vi "Get Platform.vi"(11 "Platform":T2) -> (3 "Platform":T1)   [LabVIEW 2011, in "LMH-LINX.lvlib"]
uses:
  LMH-LINX.lvlib
  Type Defs/User Platform.ctl
  Type Defs/Platform.ctl
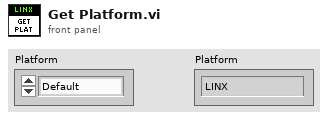
[diagram p1: front panel]
types:
  T1 = typedef "LMH-LINX.lvlib/Platform.ctl" = enum16{"LINX", "myRIO"}
  T2 = typedef "LMH-LINX.lvlib/User Platform.ctl" = enum16{"Default", "LINX", "myRIO"}
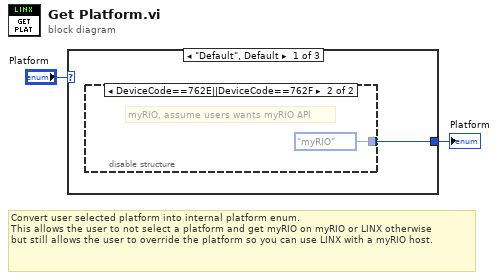
[diagram p0: block diagram]
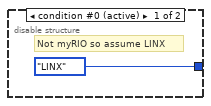
[diagram p2: hidden frame]
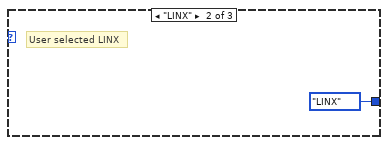
[diagram p3: hidden frame]
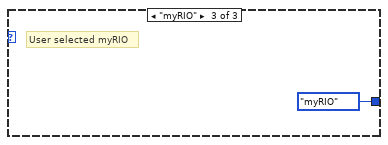
[diagram p4: hidden frame]
diagram:
  # "Convert user selected platform into internal platform enum.\nThis allows the user to not select a platform and get myRIO on myRIO or LINX otherwise\nbut still allows the user to override the platform so you can use LINX with a myRIO host."
  n1 = case shown="\"Default\", Default" "Platform" {
    tunnel: [w3 Platform."LINX" ("Platform") Platform."myRIO" ("Platform")] -> w1
    frame "Default", Default {
      n2 = disable-structure shown="DeviceCode==762E||DeviceCode==762F" {
        disable-tunnel: [Platform."LINX" ("Platform") Platform."myRIO" ("Platform")] -> w3
        frame condition #0 (active) {
          # "Not myRIO so assume LINX"
        }
        frame condition #1 {
          # "myRIO, assume users wants myRIO API"
        }
      }
    }
    frame "LINX" {
      # "User selected LINX"
    }
    frame "myRIO" {
      # "User selected myRIO"
    }
  }
  "Platform" <- w1
